vi "Flatten.vi"(6 "FIFO Timestamps":T2, 7 "Timeout (ms)":i32, 8 "error in (no error)":errorcluster, 10 "Data In":T1[](array[typedef]), 11 "CIF_NIChn_FIFO_DAQ in":refnum<class "CIF_NIChn_FIFO_DAQ_DVR.lvclass">) -> (0 "error out":errorcluster, 1 "timed out?":bool, 2 "Data Out":T1[](array[typedef]), 3 "CIF_NIChn_FIFO_DAQ out":refnum<class "CIF_NIChn_FIFO_DAQ_DVR.lvclass">, 5 "Remaining timeout (ms)":i32=100)   [LabVIEW 2021, in "CIF_NIChn_FIFO_DAQ_DVR.lvclass"]
uses:
  CIF_NIChn_FIFO_DAQ_DVR.lvclass
  CIFChannels/CIFChannels.lvclass
  587a020d-d764-4ff7-9451-6b801beca2fa.vi
  b511efe2-f594-4971-95dc-73ac55586360.vi
  D:/dev/Packages/Channel_Manager/src/CIFChannels/CIFChannels.lvclass
  ChannelCommon/typedef/TimeStamps.ctl
  ChannelCommon/ChannelCommon.lvlib
  ChannelCommon/typedef/Datatype Waveform.ctl
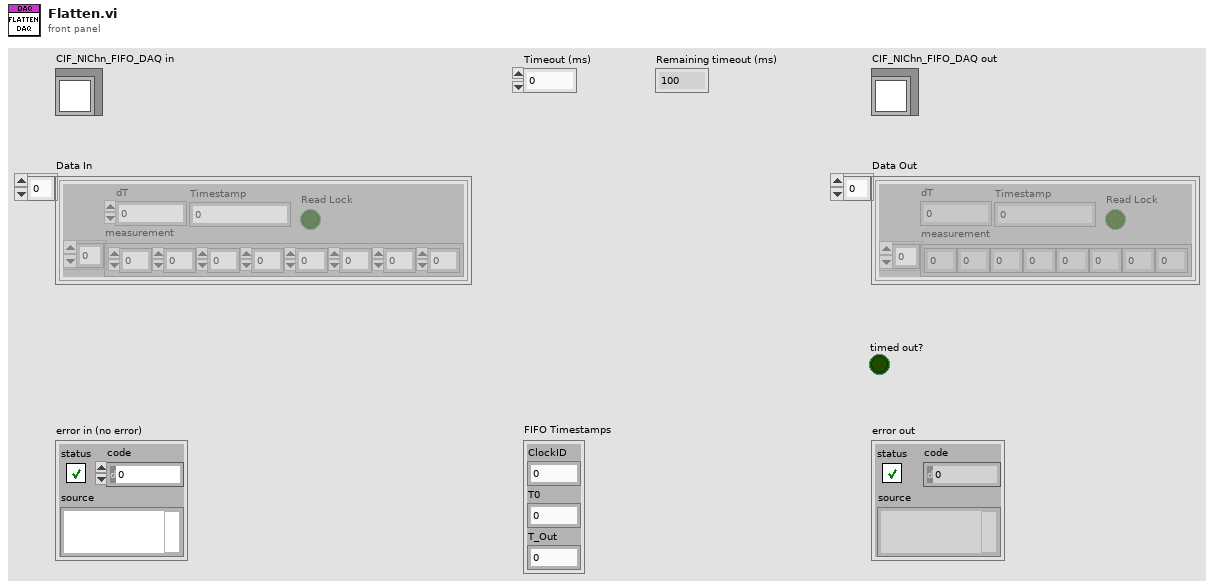
[diagram p1: front panel]
types:
  T1 = typedef "ChannelCommon.lvlib/Datatype Waveform.ctl" = cluster{"measurement":dbl[], "dT":dbl, "Timestamp":i64, "Read Lock":bool}
  T2 = typedef "ChannelCommon.lvlib/TimeStamps.ctl" = cluster{"ClockID":u8, "T0":i64, "T_Out":i64}
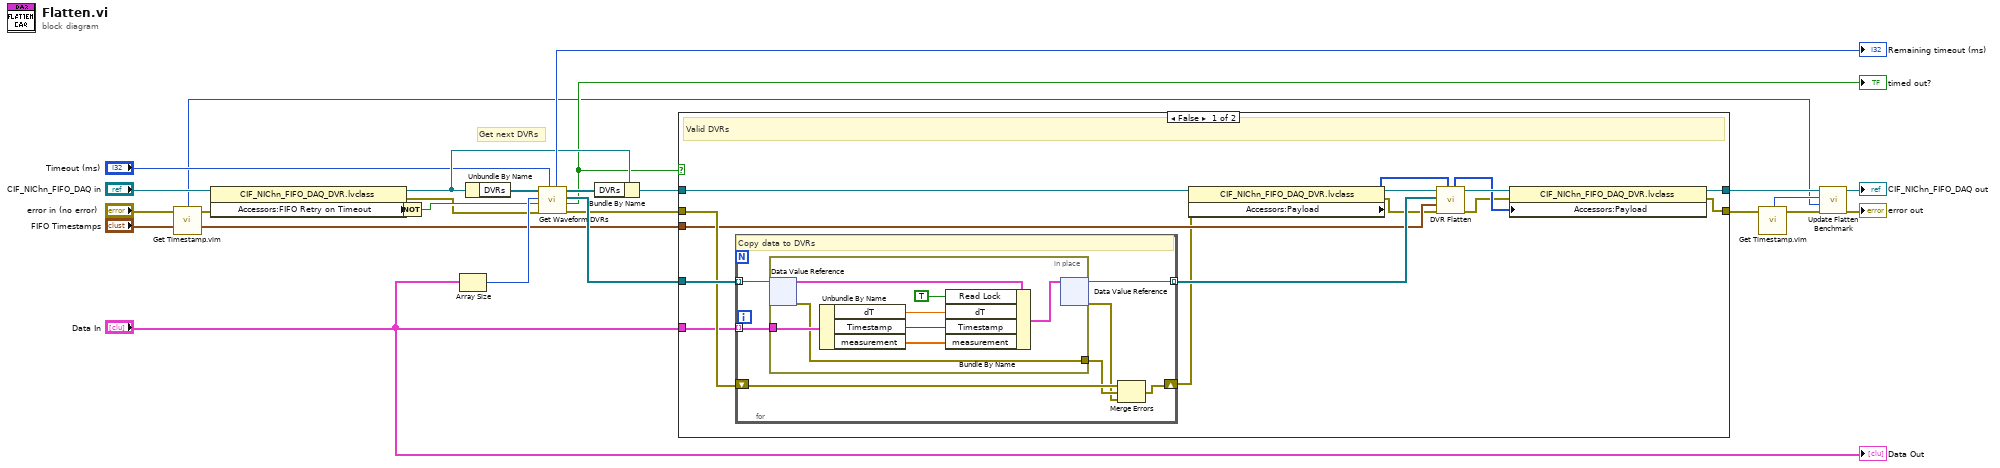
[diagram p0: block diagram]
diagram:
  # "Get next DVRs"
  n1 = call "Get Timestamp.vim"("Anything in"="error in (no error)") -> ("Time (ns)"=w1:i64, "Anything out"=w2:errorcluster)  [unwired: 2 in]
  n2 = property class="CIF_NIChn_FIFO_DAQ_DVR.lvclass"(reference="CIF_NIChn_FIFO_DAQ in", error in=w2) -> (reference out=w17:refnum<class "CIF_NIChn_FIFO_DAQ_DVR.lvclass">, error out=w15:errorcluster, "Accessors:FIFO Retry on Timeout"=w18:bool)
  n3 = Not(x=w18) -> (.not. x?=w16:bool)
  n4 = Array Size(array="Data In") -> (size(s)=w19:i32)
  n5 = Unbundle By Name(w17) -> ("DVRs"=w25:refnum<data-value>[])
  n6 = call "Get Waveform DVRs.vi"("Timeout in (ms)"="Timeout (ms)", "error in (no error)"=w15, "Ignore Read Lock"=w16, "Number of Waveforms"=w19, "DVR Circular Buffer in"=w25) -> ("error out"=w21:errorcluster, "Timeout"=w11:bool, "DVRs"=w22:refnum<data-value>[], "DVR Circular Buffer out"=w24:refnum<data-value>[], "Remaining timeout (ms)"=→"Remaining timeout (ms)":i32)  [unwired: 2 in]
  "timed out?" <- w11
  n7 = Bundle By Name(cluster=w17, "DVRs"=w24) -> (w23:refnum<class "CIF_NIChn_FIFO_DAQ_DVR.lvclass">)
  n8 = case shown="False" w11 {
    tunnel: w21 -> [w39 w56]
    tunnel: w23 -> [w35 w57]
    tunnel: w22 -> [w40 _]
    tunnel: [w28 w57] -> w9
    tunnel: [w29 w56] -> w6
    tunnel: "Data In" -> [w36 _]
    tunnel: "FIFO Timestamps" -> [w37 _]
    frame False {
      # "Valid DVRs"
      n9 = for {
        tunnel: w40 -> [w47] mode=indexing
        tunnel: w36 -> [w46] mode=indexing
        tunnel: [w45] -> w38 mode=indexing
        shift-right: [w41] -> w27
        shift-left: w39 -> [w44]
        # "Copy data to DVRs"
        n10 = in-place {
          in-place-border: w46 -> [w52]
          in-place-border: [w50] -> w43
          n11 = in-place-dvr #1(w47) -> (w55:T1, w50:errorcluster)
          n12 = Unbundle By Name(w52) -> ("dT"=w54:dbl, "Timestamp"=w53:i64, "measurement"=w48:dbl[])
          n13 = Bundle By Name(cluster=w55, "Read Lock"=TRUE, "dT"=w54, "Timestamp"=w53, "measurement"=w48) -> (w51:T1)
          n14 = in-place-dvr #1(w51) -> (w45:refnum<data-value>, w42:errorcluster)
        }
        n15 = Merge Errors(w44, w43, w42) -> (w41:errorcluster)
      }
      n16 = property class="CIF_NIChn_FIFO_DAQ_DVR.lvclass"(reference=w35, error in=w27) -> (reference out=w34:refnum<class "CIF_NIChn_FIFO_DAQ_DVR.lvclass">, error out=w26:errorcluster, "Accessors:Payload"=w33:u8[])
      n17 = call "DVR Flatten.vi"("payload in"=w33, "error in (no error)"=w26, "FIFO Timestamps"=w37, "Data In"=w38, "CIFChannels in"=w34) -> ("error out"=w30:errorcluster, "CIFChannels out"=w32:refnum<class "CIF_NIChn_FIFO_DAQ_DVR.lvclass">, "payload out"=w31:u8[])  [unwired: 2 in, 2 out]
      n18 = property class="CIF_NIChn_FIFO_DAQ_DVR.lvclass"(reference=w32, error in=w30, "Accessors:Payload"=w31) -> (reference out=w28:refnum<class "CIF_NIChn_FIFO_DAQ_DVR.lvclass">, error out=w29:errorcluster)
    }
    frame True {
      # "Timeout getting unlocked DVRs"
    }
  }
  n19 = call "Get Timestamp.vim"("Anything in"=w6) -> ("Time (ns)"=w4:i64, "Anything out"=w5:errorcluster)  [unwired: 2 in]
  n20 = call "Update Flatten Benchmark.vi"("error in (no error)"=w5, "X0"=w1, "X1"=w4, "CIFChannels in"=w9) -> ("error out"=→"error out":errorcluster, "CIFChannels out"=→"CIF_NIChn_FIFO_DAQ out":refnum<class "CIF_NIChn_FIFO_DAQ_DVR.lvclass">)  [unwired: 6 in]
  "Data Out" <- "Data In"
